vi "Cluster And Array Of Numbers.vi"(8 "Array":T1(array[cluster])=[{"Numeric"=123.0, "Numeric 2"=200, "Cluster - Level 2"={"Numeric"=789, "Array"=[4411, 5522, 3344], "Array 2"=[]}}, {"Numeric"=-12345.0, "Numeric 2"=167, "Cluster - Level 2"={"Numeric"=-2323, "Array"=[44, 55], "Array 2"=[55, 778899, 110001]}}], 9 "Cluster":T2={"Numeric"=11.0, "Numeric 2"=22, "Cluster - Level 2"={"Numeric"=33, "Array"=[44.0, 55.0]}, "Array"=[1111, 2222]}) -> ()   [LabVIEW 2011]
panel:
  in  "stop":bool
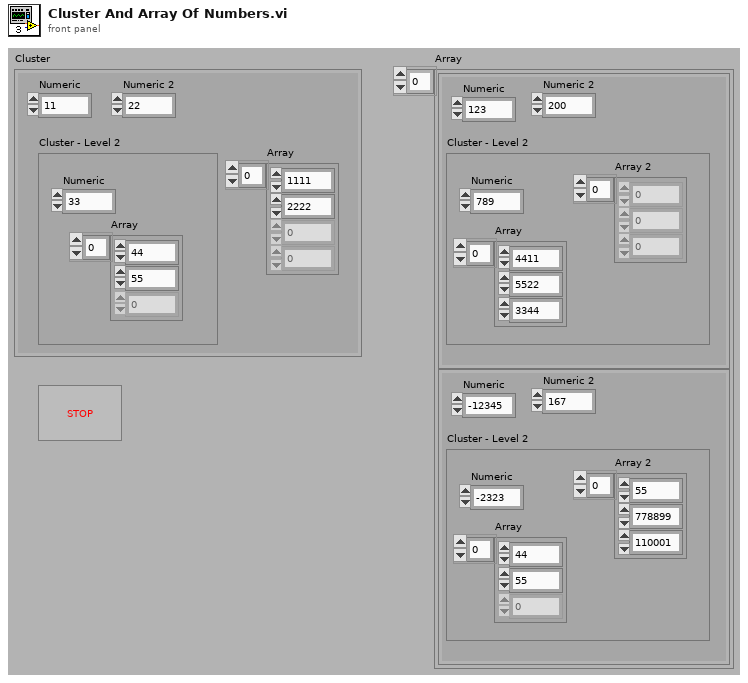
[diagram p1: front panel]
types:
  T1 = cluster{"Numeric":sgl, "Numeric 2":u8, "Cluster - Level 2":cluster{"Numeric":i16, "Array":i16[], "Array 2":u64[]}}[]
  T2 = cluster{"Numeric":dbl, "Numeric 2":i8, "Cluster - Level 2":cluster{"Numeric":u32, "Array":dbl[]}, "Array":i64[]}
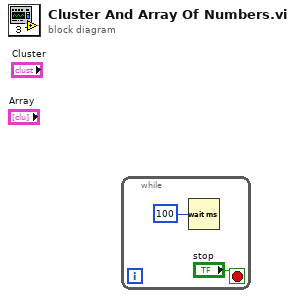
[diagram p0: block diagram]
diagram:
  n1 = while {
    stop <- "stop" stop-if-true
    n2 = Wait (ms)(milliseconds to wait=u32 100) -> ()  [unwired: 1 out]
  }
